vi "Update Motor State.vi"   [LabVIEW 2017, in "NI_Robotics_Motor Communication.lvclass"]
doc: "Writes angle or angular velocity values of the motor or motors to the motor communication session. You must manually select the polymorphic instance to use."
uses:
  <vilib>/robotics/Actuation/Motor Communication/NI_Robotics_Motor Communication.lvclass
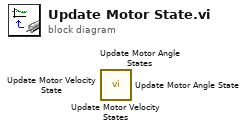
[diagram p0: block diagram]
diagram:
  n1 = call <vilib>:"Update Motor Velocity States.vi"() -> ()  [unwired: 9 in, 3 out]
  n2 = call <vilib>:"Update Motor Angle States.vi"() -> ()  [unwired: 9 in, 3 out]
  n3 = call <vilib>:"Update Motor Velocity State.vi"() -> ()  [unwired: 9 in, 3 out]
  n4 = call <vilib>:"Update Motor Angle State.vi"() -> ()  [unwired: 9 in, 3 out]
